vi "G#Object_GetAllObjectsFromSameOwner.vi"(1 "full class name (\"\")":string, 5 "error in (no error)":errorcluster) -> (12 "all refs":refnum<class "G#Object.lvclass">[](array[class]), 15 "external creator process owns":bool, 16 "no other owners":bool, 19 "error out":errorcluster)   [LabVIEW 2017, in "G#Object.lvclass"]
doc: "Returns all objects of the specified class with the same owner that called this method. If \"full class name\" is empty, all objects of all classes will be returned."
uses:
  G#Object.lvclass
  G#Object.lvclass/G#Object.ctl
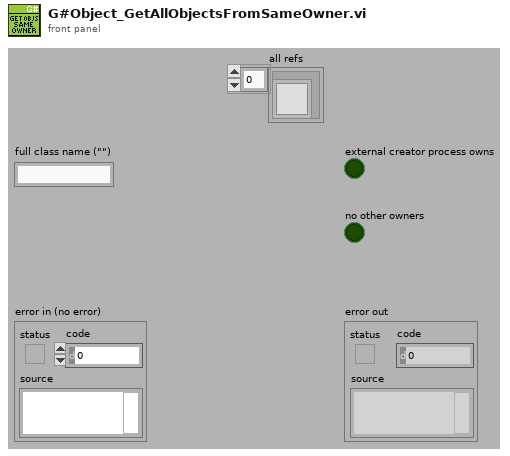
[diagram p1: front panel]
types:
  T1 = cluster{"full class name (\"\")":string, "Ref":refnum<class "G#Object.lvclass">}
  T2 = cluster{"full class name (\"\")":string, "Ref":refnum<class "G#Object.lvclass">}[]
  T3 = typedef "G#Object.lvclass/G#Object_ObjectInfoType.ctl" = cluster{"ObjectName":string, "ObjectID":u32, "Users":i32, "Counter":bool, "AttributeRefs":u32[], "FullClassName":string, "ClassName":string, "CreateMethod":T4, "GenericDestructorExists":bool, "Owner":string}
  T4 = typedef "G#Object.lvclass/G#Object_CreateMethod.ctl" = enum16{"Create", "Create or look up existing", "Look up existing"}
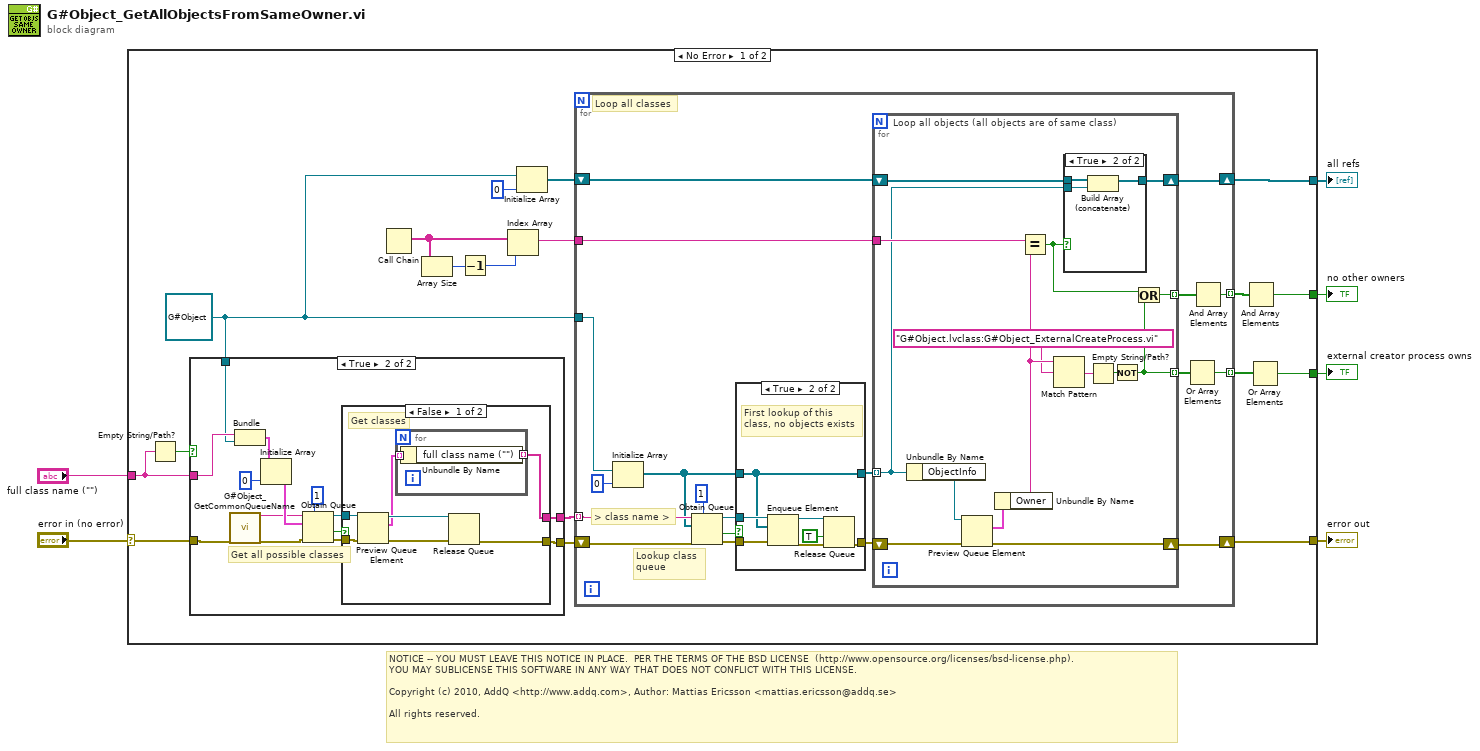
[diagram p0: block diagram]
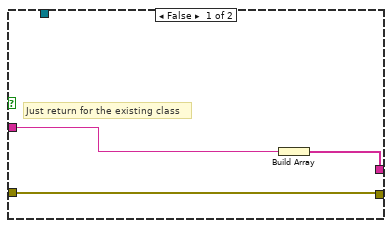
[diagram p2: hidden frame]
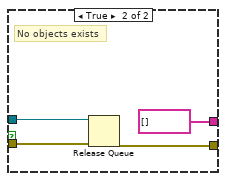
[diagram p3: hidden frame]
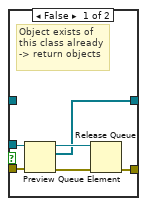
[diagram p5: hidden frame]
diagram:
  # "NOTICE -- YOU MUST LEAVE THIS NOTICE IN PLACE.  PER THE TERMS OF THE BSD LICENSE  (http://www.opensource.org/licenses/bsd-license.php).\nYOU MAY SUBLICENSE THIS SOFTWARE IN ANY WAY THAT DOES NOT CONFLICT WITH THIS LICENSE.\n\nCopyright (c) 2010, AddQ <http://www.addq.com>, Author: Mattias Ericsson <mattias.ericsson@addq.se>\n\nAll rights reserved."
  n1 = case shown="No Error" "error in (no error)" {
    selector: "error in (no error)" -> [w21 w106]
    tunnel: [w18 w106] -> w5
    tunnel: [w20 _] -> w4
    tunnel: "full class name (\"\")" -> [w16 _]
    tunnel: [w13 _] -> w2
    tunnel: [w11 _] -> w1
    frame No Error {
      w15 = refnum<class "G#Object.lvclass"> refnum ("Ref")
      n2 = Empty String/Path?(string/path=w16) -> (empty?=w17:bool)
      n3 = case shown="True" w17 {
        tunnel: [w26 w35] -> w23
        tunnel: [w27 w34] -> w22
        tunnel: w21 -> [w27 w30]
        tunnel: w16 -> [w25 w32]
        tunnel: w15 -> [_ w31]
        frame False {
          # "Just return for the existing class"
          n4 = Build Array(w25) -> (w26:string[])
        }
        frame True {
          # "Get all possible classes"
          n5 = call "G#Object_GetCommonQueueName.vi"("error in (no error)"=w30) -> ("queue name"=w28:string, "error out"=w29:errorcluster)  [unwired: 17 in]
          n6 = Bundle("full class name (\"\")"=w32, "Ref"=w31) -> (w33:T1)  [unwired: 1 in]
          n7 = Initialize Array(w33, 0 ("dimension size")) -> (w36:T2)
          n8 = Obtain Queue(max queue size (-1, unlimited)=1, name (unnamed)=w28, element data type=w36, error in (no error)=w29) -> (queue out=w39:refnum<queue>, created new?=w41:bool, error out=w40:errorcluster)  [unwired: 1 in]
          n9 = case shown="False" w41 {
            tunnel: w40 -> [w48 w51]
            tunnel: w39 -> [w47 w52]
            tunnel: [w43 string[] []] -> w35
            tunnel: [w46 w54] -> w34
            frame False {
              # "Get classes"
              n10 = Preview Queue Element(queue=w47, error in (no error)=w48) -> (queue out=w44:refnum<queue>, element=w42:T2, error out=w45:errorcluster)  [unwired: 1 in, 1 out]
              n11 = for {
                tunnel: [w50] -> w43 mode=indexing
                tunnel: w42 -> [w49] mode=indexing
                n12 = Unbundle By Name(w49) -> ("full class name (\"\")"=w50:string)
              }
              n13 = Release Queue(queue=w44, error in (no error)=w45) -> (error out=w46:errorcluster)  [unwired: 1 in, 2 out]
            }
            frame True {
              # "No objects exists"
              n14 = Release Queue(queue=w52, error in (no error)=w51) -> (error out=w54:errorcluster)  [unwired: 1 in, 2 out]
            }
          }
        }
      }
      n15 = Call Chain() -> (call chain=w10:string[])
      n16 = Array Size(array=w10) -> (size(s)=w9:i32)
      n17 = Decrement(x=w9) -> (x-1=w8:i32)
      n18 = Index Array(array=w10, index=w8) -> (element=w7:string)
      n19 = Initialize Array(w15, 0 ("dimension size")) -> (w24:refnum<class "G#Object.lvclass">[])
      n20 = for {
        shift-right: [w59] -> w18
        shift-left: w22 -> [w69]
        tunnel: w23 -> [w66] mode=indexing
        shift-right: [w60] -> w20
        shift-left: w24 -> [w62]
        tunnel: w15 -> [w65]
        tunnel: w7 -> [w61]
        tunnel: [w57] -> w14 mode=indexing
        tunnel: [w55] -> w12 mode=indexing
        # "Loop all classes"
        # "> class name >"
        # "Lookup class\nqueue"
        n21 = Initialize Array(w65, 0 ("dimension size")) -> (w64:refnum<class "G#Object.lvclass">[])
        n22 = Obtain Queue(max queue size (-1, unlimited)=1, name (unnamed)=w66, element data type=w64, error in (no error)=w69) -> (queue out=w70:refnum<queue>, created new?=w71:bool, error out=w72:errorcluster)  [unwired: 1 in]
        n23 = case shown="True" w71 {
          tunnel: w72 -> [w97 w105]
          tunnel: w70 -> [w96 w104]
          tunnel: w64 -> [_ w103]
          tunnel: [w98 w99] -> w68
          tunnel: [w93 w103] -> w67
          frame False {
            # "Object exists of\nthis class already\n-> return objects"
            n24 = Preview Queue Element(queue=w96, error in (no error)=w97) -> (queue out=w94:refnum<queue>, element=w93:refnum<class "G#Object.lvclass">[], error out=w95:errorcluster)  [unwired: 1 in, 1 out]
            n25 = Release Queue(queue=w94, error in (no error)=w95) -> (error out=w98:errorcluster)  [unwired: 1 in, 2 out]
          }
          frame True {
            # "First lookup of this\nclass, no objects exists"
            n26 = Enqueue Element(queue=w104, element=w103, error in (no error)=w105) -> (queue out=w101:refnum<queue>, error out=w100:errorcluster)  [unwired: 1 in, 1 out]
            n27 = Release Queue(queue=w101, force destroy? (F)=TRUE, error in (no error)=w100) -> (error out=w99:errorcluster)  [unwired: 2 out]
          }
        }
        n28 = for {
          shift-right: [w87] -> w59
          shift-left: w68 -> [w88]
          tunnel: w67 -> [w81] mode=indexing
          shift-right: [w82] -> w60
          shift-left: w62 -> [w83]
          tunnel: w61 -> [w84]
          tunnel: [w80] -> w58 mode=indexing
          tunnel: [w74] -> w56 mode=indexing
          # "Loop all objects (all objects are of same class)"
          n29 = Unbundle By Name(w81) -> ("ObjectInfo"=w86:refnum<queue>)
          n30 = Preview Queue Element(queue=w86, error in (no error)=w88) -> (element=w85:T3, error out=w87:errorcluster)  [unwired: 1 in, 2 out]
          n31 = Unbundle By Name(w85) -> ("Owner"=w78:string)
          n32 = Equal?(x=w84, y=w78) -> (x = y?=w79:bool)
          n33 = Match Pattern(string=w78, regular expression="G#Object.lvclass:G#Object_ExternalCreateProcess.vi") -> (match substring=w76:string)  [unwired: 1 in, 3 out]
          n34 = case shown="True" w79 {
            tunnel: w83 -> [w89 w92]
            tunnel: [w89 w91] -> w82
            tunnel: w81 -> [_ w90]
            frame False {
            }
            frame True {
              n35 = Build Array (concatenate)(w92, w90) -> (w91:refnum<class "G#Object.lvclass">[])
            }
          }
          n36 = Empty String/Path?(string/path=w76) -> (empty?=w75:bool)
          n37 = Not(x=w75) -> (.not. x?=w74:bool)
          n38 = Or(x=w79, y=w74) -> (x .or. y?=w80:bool)
        }
        n39 = Or Array Elements(Boolean array=w56) -> (logical OR=w55:bool)
        n40 = And Array Elements(Boolean array=w58) -> (logical AND=w57:bool)
      }
      n41 = And Array Elements(Boolean array=w14) -> (logical AND=w13:bool)
      n42 = Or Array Elements(Boolean array=w12) -> (logical OR=w11:bool)
    }
    frame Error {
    }
  }
  "error out" <- w5
  "all refs" <- w4
  "no other owners" <- w2
  "external creator process owns" <- w1
